vi "test12.2-AsyncMessageWithReply_Event.vi"(8 "error in (no error)":errorcluster, 11 "TestCase in":refnum<class "testcase-CSMGlobalLog.lvclass">) -> (0 "error out":errorcluster, 3 "TestCase out":refnum<class "testcase-CSMGlobalLog.lvclass">)   [LabVIEW 2017, in "testcase-CSMGlobalLog.lvclass"]
uses:
  testcase-CSMGlobalLog.lvclass
  testcase-CSMGlobalLog.lvclass/testcase-CSMGlobalLog.ctl
  src/user.lib/_NEVSTOP/Communicable State Machine(CSM)/_Support/Typedef/_CSM_GlobalLog_MSG.ctl
  src/user.lib/_NEVSTOP/Communicable State Machine(CSM)/_Support/Typedef/_CSM_Response Source Message.ctl
  src/user.lib/_NEVSTOP/Communicable State Machine(CSM)/_Support/Typedef/_CSM_GlobalLog_MSG_TYPE.ctl
  c0dc643a-0362-49fc-99f4-5251266ba5a0.vi
  src/user.lib/_NEVSTOP/Communicable State Machine(CSM)/_Support/GlobalEvent/GEvt-Generate with Rule Check.vi
  src/user.lib/_NEVSTOP/Communicable State Machine(CSM)/AdvanceAPI/CSM - Convert Error to Argument.vi
  src/user.lib/_NEVSTOP/Communicable State Machine(CSM)/AdvanceAPI/CSM - Make String Arguments Safe.vi
  src/user.lib/_NEVSTOP/Communicable State Machine(CSM)/AdvanceAPI/CSM - Keywords.vi
  src/user.lib/_NEVSTOP/Communicable State Machine(CSM)/_Support/GlobalEvent/Cache-GEvt Refs.vi
  src/user.lib/_NEVSTOP/Communicable State Machine(CSM)/_Support/GlobalEvent/LogFilter/LogFilter - Check.vi
  src/user.lib/_NEVSTOP/Communicable State Machine(CSM)/_Support/GlobalEvent/LogFilter/LogFilter.lvclass
  <vilib>/addons/_JKI Toolkits/VI Tester/TestCase.llb/TestCase.lvclass
  src/user.lib/_NEVSTOP/Communicable State Machine(CSM)/Communicable State Machine.lvlib
  C:/Program Files (x86)/National Instruments/LabVIEW 2017/vi.lib/addons/_JKI Toolkits/VI Tester/TestCase.llb/TestCase.lvclass
panel:
  out "String cache each loop":string
  out "error out 2":errorcluster
  out "Timed out":bool[](array[boolean])
  out "LoopCount":i32
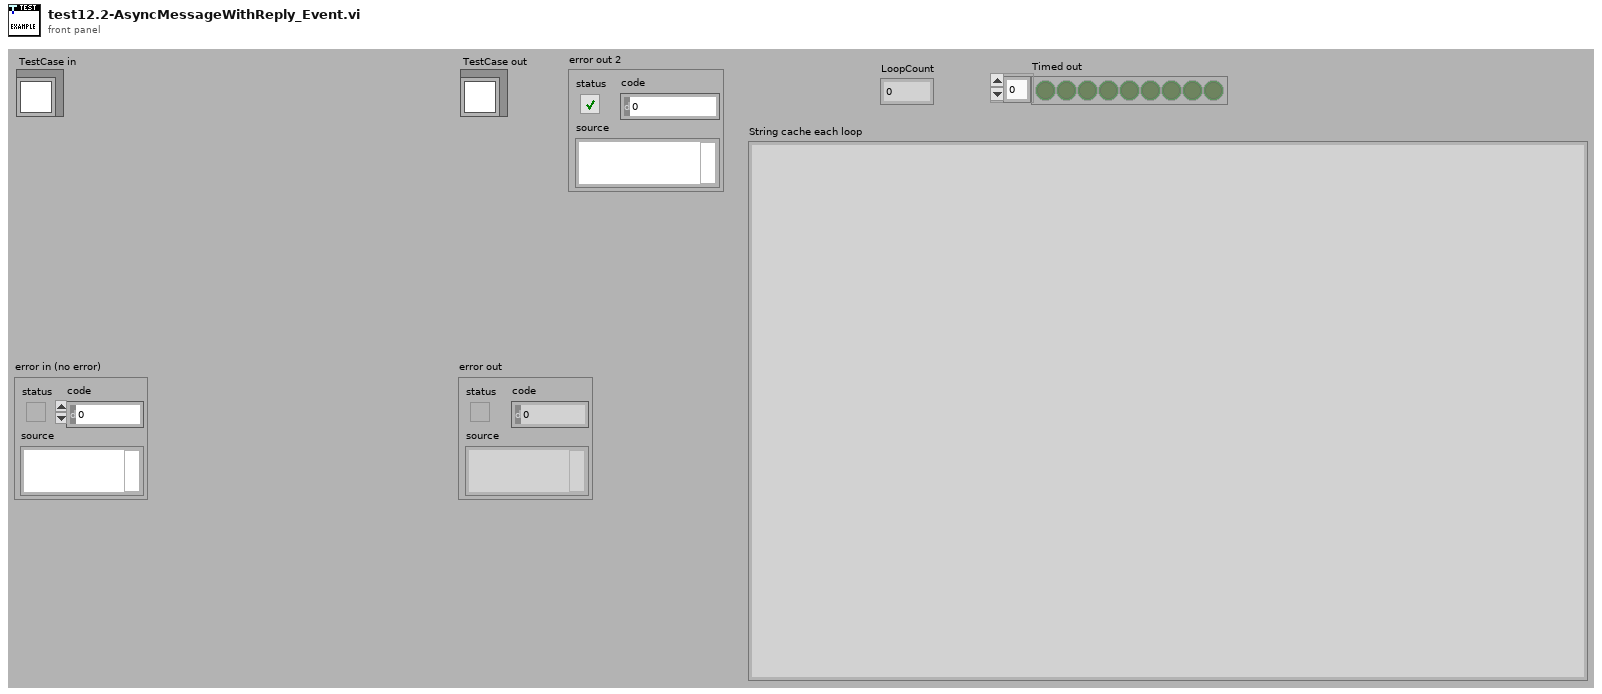
[diagram p1: front panel]
types:
  T1 = typedef "Communicable State Machine.lvlib/_CSM_GlobalLog_MSG.ctl" = cluster{"Name (\"\" to Use UUID)":string, "Current State":string, "Arguments":string, "Source Message":T2, "Source Module":string, "Complete(T)/Start(F)":bool, "LogType":T3, "Time Stamp":timestamp}
  T2 = typedef "Communicable State Machine.lvlib/_CSM_Response Source Message.ctl" = cluster{"‘State":string, "’Arguments":string, "’Error":errorcluster}
  T3 = typedef "Communicable State Machine.lvlib/_CSM_GlobalLog_MSG_TYPE.ctl" = enum16{"User Log", "State Change", "Status", "Interrupt", "Register", "Unregister", "Error Log", "Module Created", "Module Destroyed", "Async Message", "No-Rep Async Message", "Sync Message"}
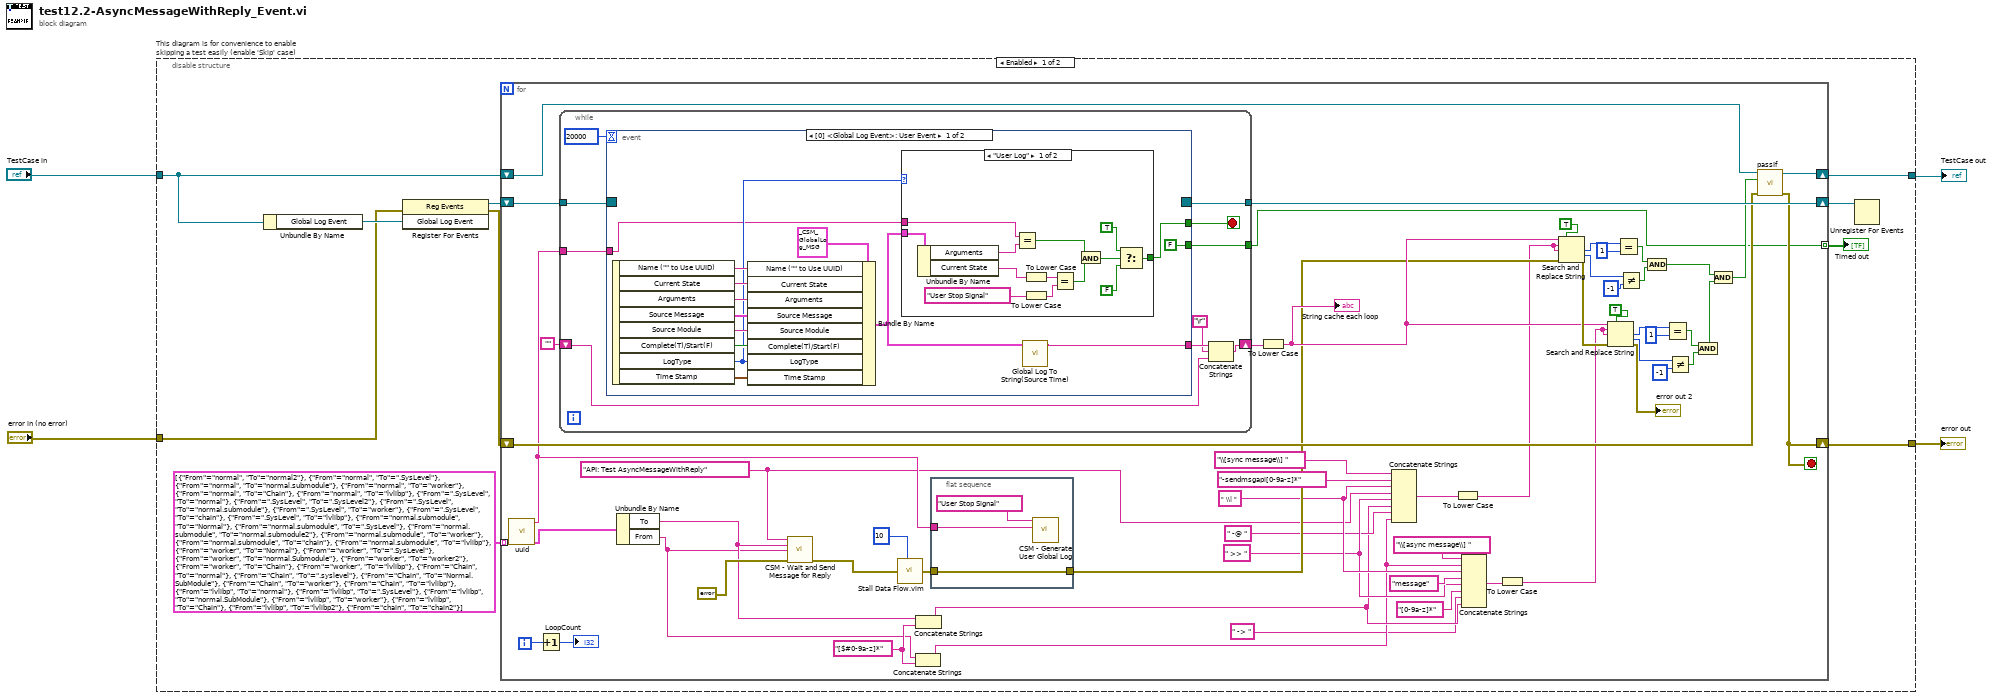
[diagram p0: block diagram]
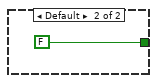
[diagram p2: hidden frame]
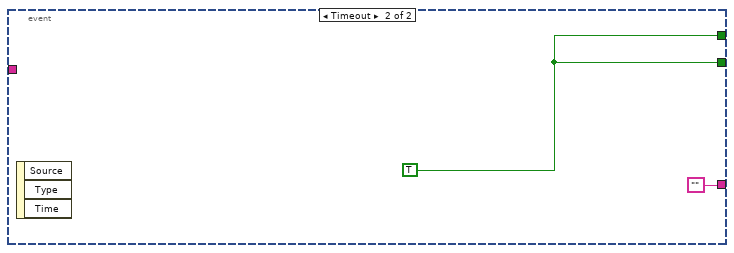
[diagram p3: hidden frame]
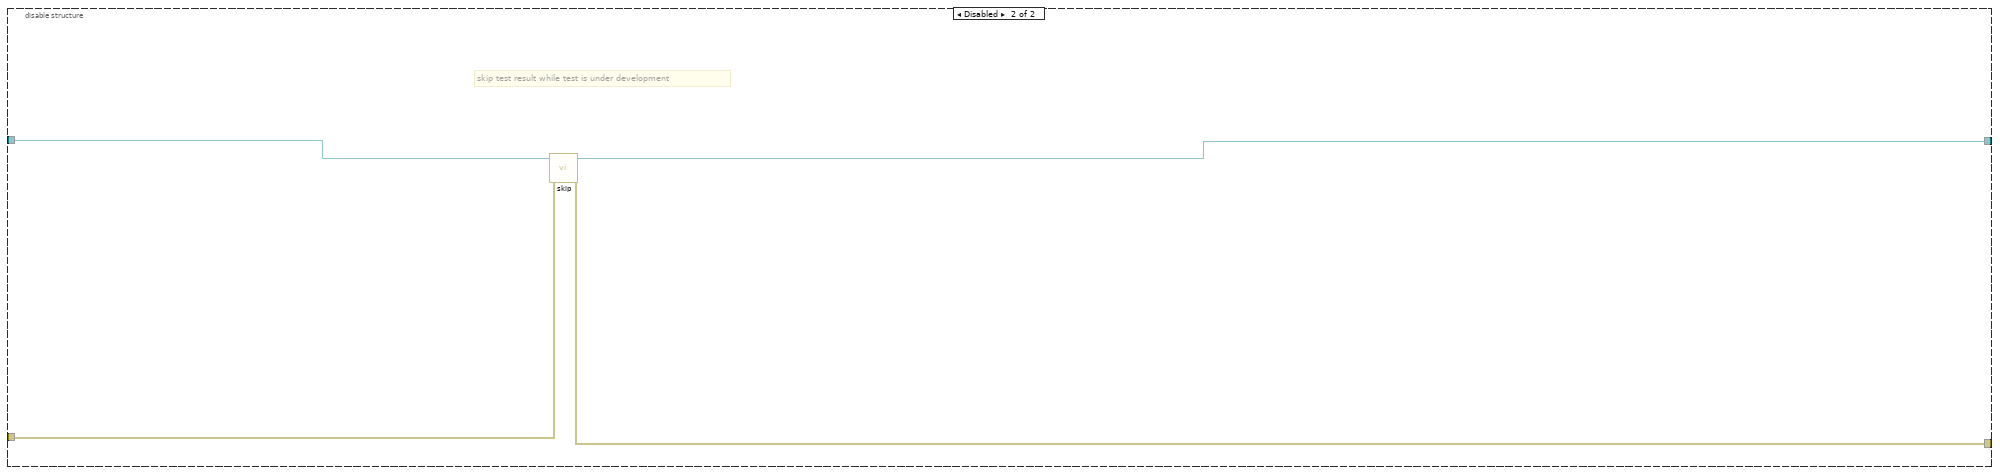
[diagram p4: hidden frame]
diagram:
  n1 = disable-structure "This diagram is for convenience to enable skipping a test easily (enable 'Skip' case)" shown="Enabled" {
    disable-tunnel: "TestCase in" -> [w9 w118]
    disable-tunnel: [w8 w116] -> w1
    disable-tunnel: [w7 w117] -> w3
    disable-tunnel: "error in (no error)" -> [w13 w115]
    frame Enabled {
      n2 = Unbundle By Name(w9) -> ("Global Log Event"=w14:refnum<user-event>)
      n3 = register-events(error in=w13, w14) -> (reference out=w12:refnum<event-registration>, error out=w10:errorcluster)  [unwired: 1 in]
      n4 = for {
        shift-right: [w70] -> w11
        shift-left: w12 -> [w71]
        shift-right: [w66] -> w7
        shift-left: w10 -> [w68]
        tunnel: cluster{"From":string, "To":string}[] [{"From"="normal", "To"="normal2"}, {"From"="normal", "To"=".SysLevel"}, {"From"="normal", "To"="normal.submodule"}, {"From"="normal", "To"="worker"}, {"From"="normal", "To"="Chain"}, {"From"="normal", "To"="lvlibp"}, {"From"=".SysLevel", "To"="normal"}, {"From"=".SysLevel", "To"=".SysLevel2"}, {"From"=".SysLevel", "To"="normal.submodule"}, {"From"=".SysLevel", "To"="worker"}, {"From"=".SysLevel", "To"="chain"}, {"From"=".SysLevel", "To"="lvlibp"}, {"From"="normal.submodule", "To"="Normal"}, {"From"="normal.submodule", "To"=".SysLevel"}, {"From"="normal.submodule", "To"="normal.submodule2"}, {"From"="normal.submodule", "To"="worker"}, {"From"="normal.submodule", "To"="chain"}, {"From"="normal.submodule", "To"="lvlibp"}, {"From"="worker", "To"="Normal"}, {"From"="worker", "To"=".SysLevel"}, {"From"="worker", "To"="normal.Submodule"}, {"From"="worker", "To"="worker2"}, {"From"="worker", "To"="Chain"}, {"From"="worker", "To"="lvlibp"}, {"From"="Chain", "To"="normal"}, {"From"="Chain", "To"=".syslevel"}, {"From"="Chain", "To"="Normal.SubModule"}, {"From"="Chain", "To"="worker"}, {"From"="Chain", "To"="lvlibp"}, {"From"="lvlibp", "To"="normal"}, {"From"="lvlibp", "To"=".SysLevel"}, {"From"="lvlibp", "To"="normal.SubModule"}, {"From"="lvlibp", "To"="worker"}, {"From"="lvlibp", "To"="Chain"}, {"From"="lvlibp", "To"="lvlibp2"}, {"From"="chain", "To"="chain2"}] -> [w45] mode=indexing
        shift-right: [w69] -> w8
        shift-left: w9 -> [w65]
        tunnel: [w34] -> w5 mode=indexing
        i -> [w42]
        stop <- w66 stop-if-true
        w21 = "[$#0-9a-z]*" ("string")
        w29 = " >> "
        w31 = " \\| "
        w24 = "API: Test AsyncMessageWithReply" ("State")
        n5 = call "uuid.vi"() -> ("UUID"=w43:string)  [unwired: 11 in]
        n6 = Increment(x=w42) -> (x+1=→"LoopCount":i32)
        n7 = while {
          tunnel: w71 -> [w84]
          tunnel: [w83] -> w70
          shift-right: [w75] -> w35
          shift-left: "" -> [w78]
          tunnel: w43 -> [w80]
          tunnel: [w79] -> w34
          stop <- w82 stop-if-true
          n8 = event shown="[0] <Global Log Event>: User Event" {
            selector: w84 -> [_ _]
            dyn-events: [_ _] -> w83
            timeout: 20000 -> [_ _]
            tunnel: [w85 ""] -> w77
            tunnel: [w87 w114] -> w82
            tunnel: w80 -> [w88 _]
            tunnel: [FALSE ("Stop") w114] -> w79
            event User Event {
              n9 = event-data() -> ("Name (\"\" to Use UUID)"=w97:string, "Current State"=w96:string, "Arguments"=w95:string, "Source Message"=w94:T2, "Source Module"=w93:string, "Complete(T)/Start(F)"=w92:bool, "LogType"=w89:T3, "Time Stamp"=w91:timestamp)  [unwired: 1 in]
              n10 = Bundle By Name(cluster=T1 {"Name (\"\" to Use UUID)"="", "Current State"="", "Arguments"="", "Source Message"={"‘State"="", "’Arguments"="", "’Error"={"status"=FALSE, "code"=0, "source"=""}}, "Source Module"="", "Complete(T)/Start(F)"=FALSE, "LogType"=enum."State Change", "Time Stamp"=timestamp(0 s since 1904-01-01)} ("Cross CSM Data"), "Name (\"\" to Use UUID)"=w97, "Current State"=w96, "Arguments"=w95, "Source Message"=w94, "Source Module"=w93, "Complete(T)/Start(F)"=w92, "LogType"=w89, "Time Stamp"=w91) -> (w86:T1)
              n11 = case shown="\"User Log\"" w89 {
                tunnel: w86 -> [w111 _]
                tunnel: w88 -> [w110 _]
                tunnel: [w99 FALSE] -> w87
                frame "User Log" {
                  n12 = Unbundle By Name(w111) -> ("Arguments"=w109:string, "Current State"=w108:string)
                  n13 = Equal?(x=w110, y=w109) -> (x = y?=w103:bool)
                  n14 = To Lower Case(string=w108) -> (all lower case string=w107:string)
                  n15 = To Lower Case(string="User Stop Signal" ("Log")) -> (all lower case string=w105:string)
                  n16 = Equal?(x=w107, y=w105) -> (x = y?=w104:bool)
                  n17 = And(x=w103, y=w104) -> (x .and. y?=w102:bool)
                  n18 = Select(t=TRUE, s=w102, f=FALSE) -> (s? t:f=w99:bool)
                }
                frame Default {
                }
              }
              n19 = call "Global Log To String(Source Time).vi"("Log"=w86) -> ("Log String"=w85:string)  [unwired: 9 in]
            }
            event Timeout {
              w114 = TRUE ("Stop")
              n20 = event-data() -> ()  [unwired: 1 in, 3 out]
            }
          }
          n21 = Concatenate Strings(w77, "\r", w78) -> (w75:string)
        }
        n22 = Unbundle By Name(w45) -> ("To"=w20:string, "From"=w19:string)
        n23 = call "CSM - Wait and Send Message for Reply.vi"("State"=w24, "Arguments (\"\")"=w20, "Target Module"=w19, "Error In (No Error)"=errorcluster {"status"=FALSE, "code"=0, "source"=""} ("error out")) -> ("error out"=w39:errorcluster)  [unwired: 9 in, 2 out]
        n24 = call "Stall Data Flow.vim"("value in"=w39, "milliseconds to wait"=u32 10) -> ("value out"=w44:errorcluster)  [unwired: 1 out]
        n25 = Concatenate Strings(w19, w21) -> (w17:string)
        n26 = Concatenate Strings(w20, w21) -> (w18:string)
        n27 = flat-sequence {
          tunnel: w43 -> [w73]
          tunnel: w44 -> [w72]
          tunnel: [w72] -> w36
          frame #0 {
            n28 = call "CSM - Generate User Global Log.vi"("Arguments"=w73, "Log"="User Stop Signal") -> ()  [unwired: 9 in, 1 out]
          }
        }
        n29 = To Lower Case(string=w35) -> (all lower case string=w37:string)
        "String cache each loop" <- w37
        n30 = Concatenate Strings("\\[sync message\\] ", "-sendmsgapi[0-9a-z]*", w31, w24, w29, w18, " -@ ", w17) -> (w26:string)
        n31 = To Lower Case(string=w26) -> (all lower case string=w23:string)
        n32 = Concatenate Strings("\\[async message\\] " ("string"), w17, w31, "message", w29, "[0-9a-z]*", " -> ", w18) -> (w25:string)
        n33 = To Lower Case(string=w25) -> (all lower case string=w22:string)
        n34 = Search and Replace String(replace all?=TRUE ("replace all? (F)"), input string=w37, search string=w23, replace string=w23, error in=w36) -> (number of replacements=w53:i32, offset past replacement=w54:i32, error out=w61:errorcluster)  [unwired: 3 in, 1 out]
        n35 = Search and Replace String(replace all?=TRUE ("replace all? (F)"), input string=w37, search string=w22, replace string=w22, error in=w61) -> (number of replacements=w60:i32, offset past replacement=w59:i32, error out=→"error out 2":errorcluster)  [unwired: 3 in, 1 out]
        n36 = Equal?(x=w53, y=1) -> (x = y?=w55:bool)
        n37 = Not Equal?(x=w54, y=-1) -> (x != y?=w56:bool)
        n38 = And(x=w55, y=w56) -> (x .and. y?=w64:bool)
        n39 = Equal?(x=w60, y=1) -> (x = y?=w58:bool)
        n40 = Not Equal?(x=w59, y=-1) -> (x != y?=w57:bool)
        n41 = And(x=w58, y=w57) -> (x .and. y?=w62:bool)
        n42 = And(x=w64, y=w62) -> (x .and. y?=w41:bool)
        n43 = call-dynamic "passIf.vi"("error in (no error)"=w68, "pass"=w41, "TestCase in"=w65) -> ("error out"=w66:errorcluster, "TestCase out"=w69:refnum<class "testcase-CSMGlobalLog.lvclass">)  [unwired: 7 in]
      }
      "Timed out" <- w5
      n44 = Unregister For Events(event registration refnum=w11) -> ()  [unwired: 1 in, 1 out]
    }
    frame Disabled {
      # "skip test result while test is under development"
      n45 = call <vilib>:"skip.vi"("error in (no error)"=w115, "TestCase in"=w118) -> ("error out"=w117:errorcluster, "TestCase out"=w116:refnum<class "testcase-CSMGlobalLog.lvclass">)  [unwired: 8 in]
    }
  }
  "error out" <- w3
  "TestCase out" <- w1
